vi "Write Threshold Boundaries.vi"(8 "error in (no error)":errorcluster, 10 "Threshold Boundaries":cluster{"Minimum":dbl, "Maximum":dbl}, 11 "Video Processor in":refnum<class "Video Cam Processor.lvclass">) -> (0 "error out":errorcluster, 3 "Video Processor out":refnum<class "Video Cam Processor.lvclass">)   [LabVIEW 2018, in "Video Cam Processor.lvclass"]
uses:
  Video Cam Processor.lvclass
  Video Cam Processor.lvclass/Video Cam Processor.ctl
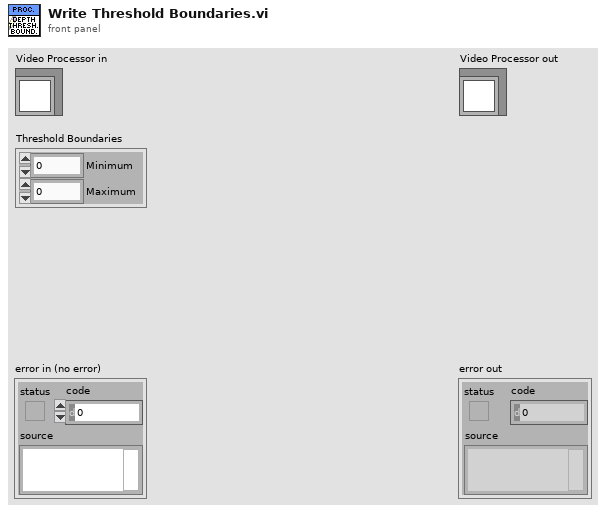
[diagram p1: front panel]
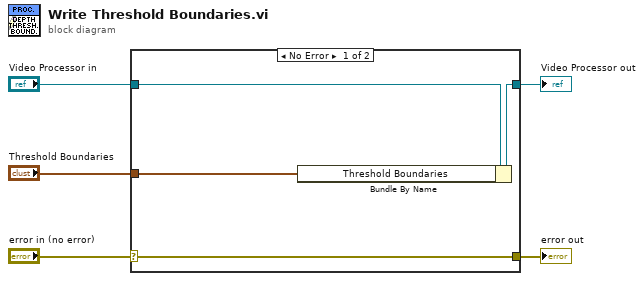
[diagram p0: block diagram]
diagram:
  n1 = case shown="No Error" "error in (no error)" {
    selector: "error in (no error)" -> [w9 w10]
    tunnel: [w9 w10] -> w4
    tunnel: [w7 w11] -> w2
    tunnel: "Video Processor in" -> [w8 w11]
    tunnel: "Threshold Boundaries" -> [w6 _]
    frame No Error {
      n2 = Bundle By Name(cluster=w8, "Threshold Boundaries"=w6) -> (w7:refnum<class "Video Cam Processor.lvclass">)
    }
    frame Error {
    }
  }
  "error out" <- w4
  "Video Processor out" <- w2
